vi "element_is_edge.vi"(10 "current element":i16, 11 "edge_cluster":cluster{"Array":sgl[], "Array":bool[]}) -> (2 "direction (rising/falling)":bool, 3 "edge":bool)   [LabVIEW 2011]
panel:
  out "Boolean":bool
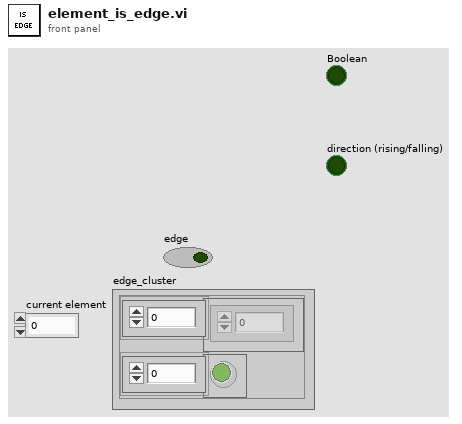
[diagram p1: front panel]
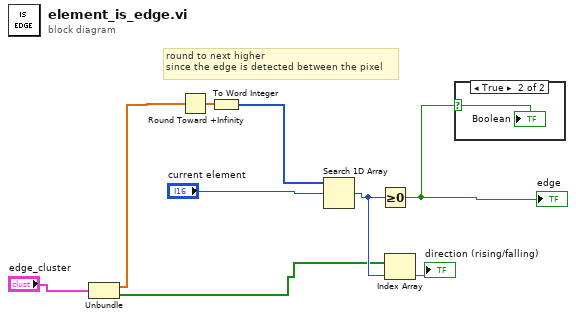
[diagram p0: block diagram]
diagram:
  # "round to next higher \nsince the edge is detected between the pixel"
  n1 = Unbundle("edge_cluster") -> ("Array"=w4:sgl[], "Array"=w3:bool[])
  n2 = Round Toward +Infinity(x=w4) -> (ceil(x): smallest int >= x=w8:sgl[])
  n3 = To Word Integer(number=w8) -> (16bit integer=w7:i16[])
  n4 = Search 1D Array(1D array=w7, element="current element") -> (index of element=w6:i32)  [unwired: 1 in]
  n5 = Greater Or Equal To 0?(x=w6) -> (x >= 0?=w1:bool)
  "edge" <- w1
  n6 = Index Array(array=w3, index=w6) -> (element=→"direction (rising/falling)":bool)
  n7 = case shown="True" w1 {
    selector: w1 -> [_ w10]
    frame False {
    }
    frame True {
      "Boolean" <- w10
    }
  }
